vi "Set State Connections.vi"(8 "error in":errorcluster, 9 "connections":T1[](array[typedef]), 10 "state":string, 11 "routing channel in":T2 format="%.0x") -> (0 "error out":errorcluster, 3 "routing channel out":T2=18446744073709551615 format="%.0x")   [LabVIEW 2017, in "Routing and Faulting Scripting.lvlib"]
uses:
  Routing and Faulting Scripting.lvlib
  <vilib>/NI Veristand/Custom Device API/Custom Device Item Ref.ctl
  Shared/Connection.ctl
  Shared/Routing and Faulting Shared.lvlib
  <vilib>/NI Veristand/Custom Device API/Custom Device API.lvlib
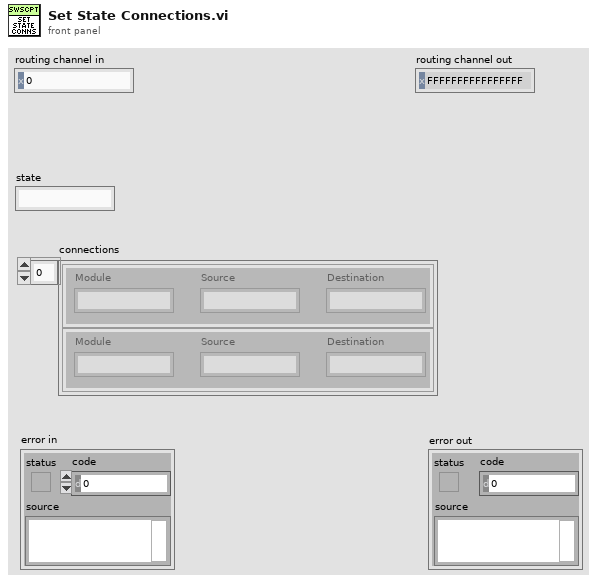
[diagram p1: front panel]
types:
  T1 = typedef "Routing and Faulting Shared.lvlib/Connection.ctl" = cluster{"Module":string, "Source":string, "Destination":string}
  T2 = typedef "Custom Device API.lvlib/Custom Device Item Ref.ctl" = u64
  T3 = typedef "Routing and Faulting Shared.lvlib/Routing State.ctl" = cluster{"Name":string, "Description":string, "Value":i32, "Connection List":T1[]}
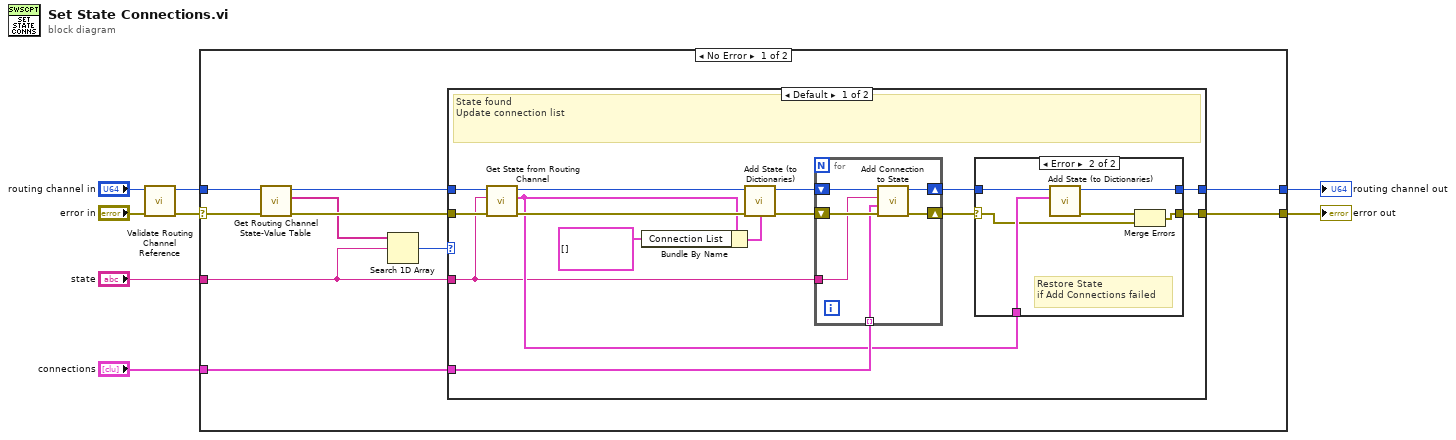
[diagram p0: block diagram]
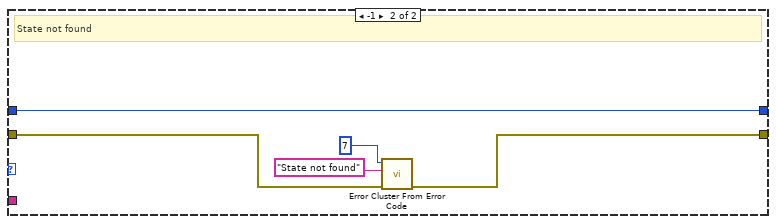
[diagram p3: hidden frame]
diagram:
  n1 = call "Validate Routing Channel Reference.vi"("error in (no error)"="error in", "Channel Ref in"="routing channel in") -> ("error out"=w3:errorcluster, "Channel Ref out"=w1:T2)  [unwired: 8 in]
  n2 = case shown="No Error" w3 {
    selector: w3 -> [w17 w54]
    tunnel: [w13 w54] -> w4
    tunnel: w1 -> [w18 w53]
    tunnel: [w14 w53] -> w5
    tunnel: "state" -> [w11 _]
    tunnel: "connections" -> [w9 _]
    frame No Error {
      n3 = call "Get Routing Channel State-Value Table.vi"("error in"=w17, "routing channel in"=w18) -> ("error out"=w15:errorcluster, "state names"=w12:string[], "routing channel out"=w16:T2)  [unwired: 6 in, 1 out]
      n4 = Search 1D Array(1D array=w12, element=w11) -> (index of element=w10:i32)  [unwired: 1 in]
      n5 = case shown="Default" w10 {
        tunnel: w16 -> [w33 w49]
        tunnel: w15 -> [w32 w51]
        tunnel: [w23 w49] -> w14
        tunnel: [w25 w50] -> w13
        tunnel: w11 -> [w19 _]
        tunnel: w9 -> [w21 _]
        frame Default {
          # "State found\nUpdate connection list"
          n6 = call "Get State from Routing Channel.vi"("error in"=w32, "state"=w19, "routing channel in"=w33) -> ("error out"=w29:errorcluster, "state and connections"=w20:T3, "routing channel out"=w31:T2)  [unwired: 6 in]
          n7 = Bundle By Name(cluster=w20, "Connection List"=T1[] []) -> (w28:T3)
          n8 = call "Add State (to Dictionaries).vi"("error in"=w29, "state and connections"=w28, "routing channel in"=w31) -> ("error out"=w30:errorcluster, "routing channel out"=w26:T2)  [unwired: 7 in]
          n9 = for {
            shift-right: [w46] -> w22
            shift-left: w30 -> [w47]
            shift-right: [w44] -> w24
            shift-left: w26 -> [w45]
            tunnel: w19 -> [w43]
            tunnel: w21 -> [w42] mode=indexing
            n10 = call "Add Connection to State.vi"("error in"=w47, "connection"=w42, "state"=w43, "routing channel in"=w45) -> ("error out"=w46:errorcluster, "routing channel out"=w44:T2)  [unwired: 6 in]
          }
          n11 = case shown="Error" w22 {
            selector: w22 -> [w35 w37]
            tunnel: [w35 w36] -> w25
            tunnel: w24 -> [w34 w41]
            tunnel: [w34 w40] -> w23
            tunnel: w20 -> [_ w39]
            frame No Error {
            }
            frame Error {
              # "Restore State\nif Add Connections failed"
              n12 = call "Add State (to Dictionaries).vi"("state and connections"=w39, "routing channel in"=w41) -> ("error out"=w38:errorcluster, "routing channel out"=w40:T2)  [unwired: 8 in]
              n13 = Merge Errors(w38, w37) -> (w36:errorcluster)
            }
          }
        }
        frame -1 {
          # "State not found"
          n14 = call <vilib>:"Error Cluster From Error Code.vi"("error in (no error)"=w51, "error message (\"\")"="State not found" ("error message (\"\")"), "error code (0)"=7) -> ("error out"=w50:errorcluster)  [unwired: 6 in]
        }
      }
    }
    frame Error {
    }
  }
  "routing channel out" <- w5
  "error out" <- w4
